vi "ROI.vi"(0 "input cluster":T2) -> (1 "Acquired Buffer Number":u32, 2 "Output First-call":bool=TRUE, 3 "Output ROI Array":dbl[][](array[numeric]))   [LabVIEW 2010]
uses:
  <vilib>/userDefined/High Color/IMAQdx.ctl
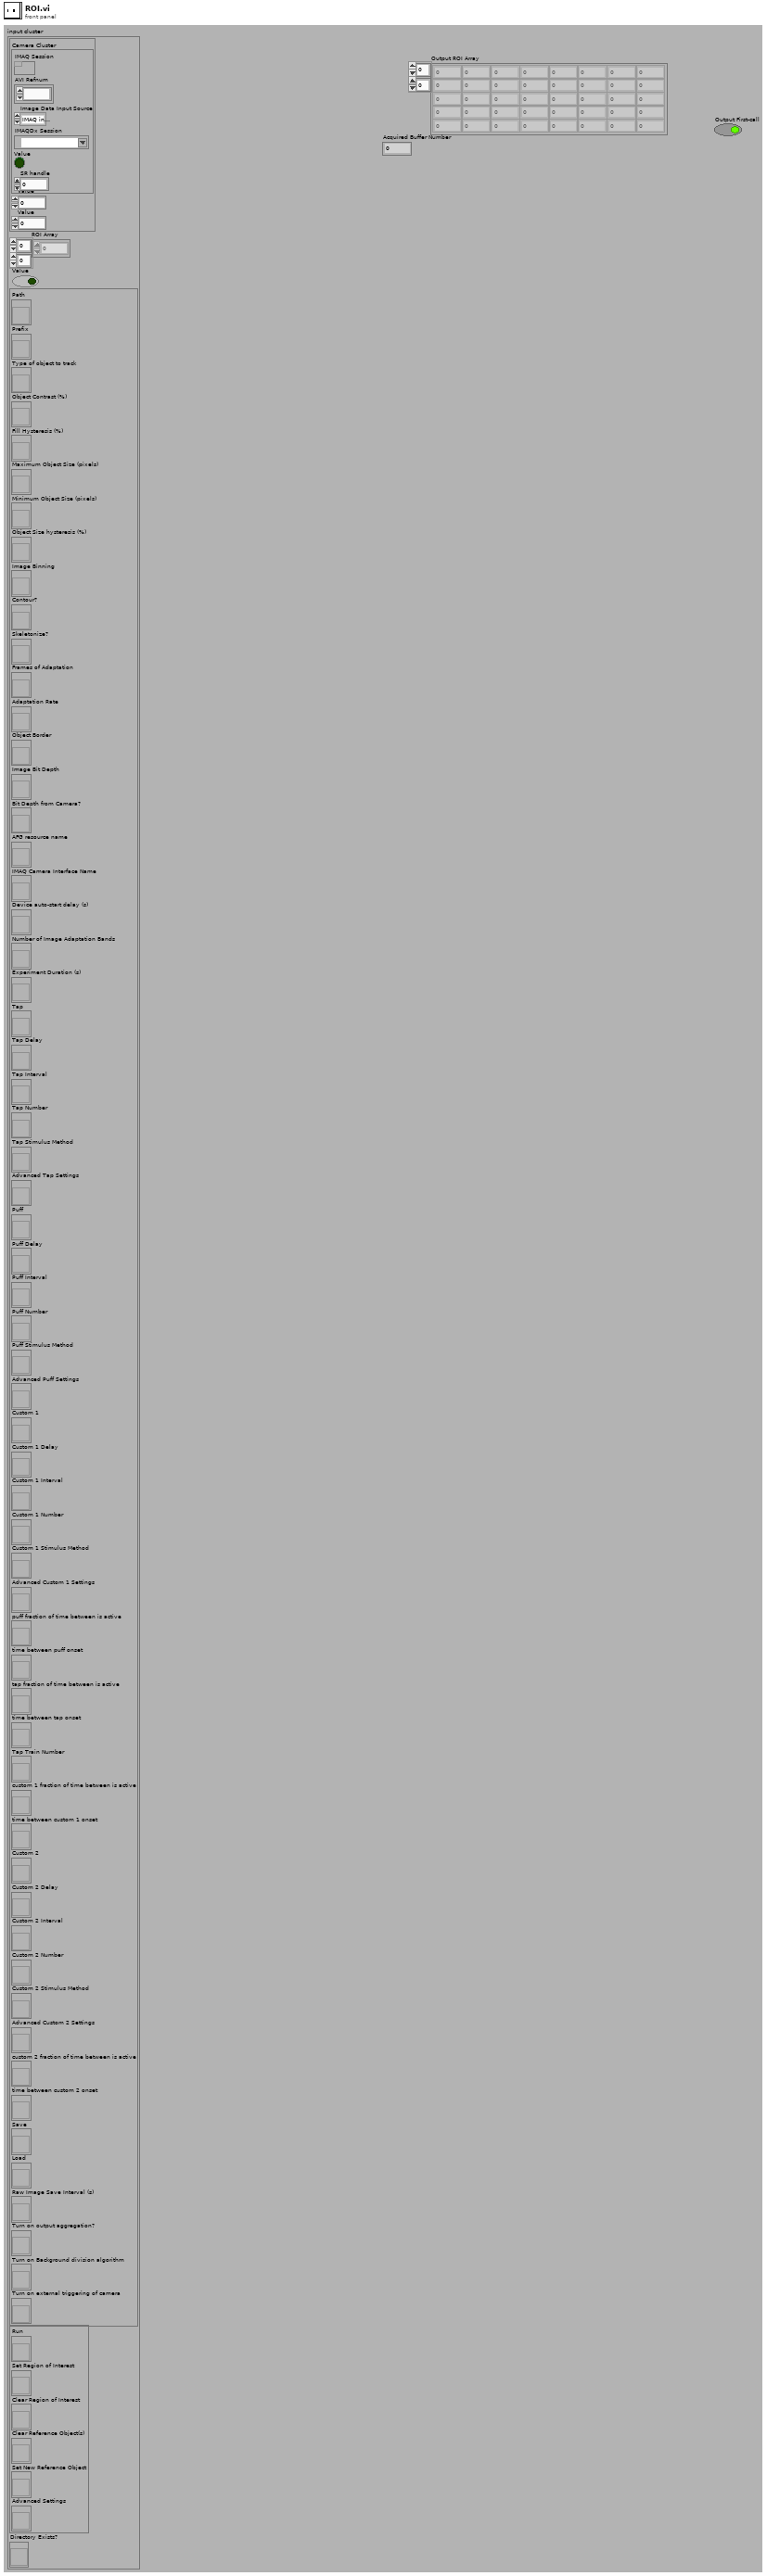
[diagram p1: front panel]
types:
  T1 = typedef "IMAQdx.ctl" = refnum<k21>
  T2 = cluster{cluster{"Camera Cluster":cluster{"IMAQ Session":refnum<k11>, "AVI Refnum":refnum<k1>, "Image Data Input Source":enum32{"IMAQ interface", "IMAQdx interface", "AVI file", "MMF File"}, "IMAQDx Session":T1, "Value":bool, "SR handle":u32}, "Value":i32, "Value":i32}, "ROI Array":dbl[][], "Value":bool, cluster{"Path":refnum<vi>, "Prefix":refnum<vi>, "Type of object to track":refnum<vi>, "Object Contrast (%)":refnum<vi>, "Fill Hysteresis (%)":refnum<vi>, "Maximum Object Size (pixels)":refnum<vi>, "Minimum Object Size (pixels)":refnum<vi>, "Object Size hysteresis (%)":refnum<vi>, "Image Binning":refnum<vi>, "Contour?":refnum<vi>, "Skeletonize?":refnum<vi>, "Frames of Adaptation":refnum<vi>, "Adaptation Rate":refnum<vi>, "Object Border":refnum<vi>, "Image Bit Depth":refnum<vi>, "Bit Depth from Camera?":refnum<vi>, "AFG resource name":refnum<vi>, "IMAQ Camera Interface Name":refnum<vi>, "Device auto-start delay (s)":refnum<vi>, "Number of Image Adaptation Bands":refnum<vi>, "Experiment Duration (s)":refnum<vi>, "Tap":refnum<vi>, "Tap Delay":refnum<vi>, "Tap Interval":refnum<vi>, "Tap Number":refnum<vi>, "Tap Stimulus Method":refnum<vi>, "Advanced Tap Settings":refnum<vi>, "Puff":refnum<vi>, "Puff Delay":refnum<vi>, "Puff Interval":refnum<vi>, "Puff Number":refnum<vi>, "Puff Stimulus Method":refnum<vi>, "Advanced Puff Settings":refnum<vi>, "Custom 1":refnum<vi>, "Custom 1 Delay":refnum<vi>, "Custom 1 Interval":refnum<vi>, "Custom 1 Number":refnum<vi>, "Custom 1 Stimulus Method":refnum<vi>, "Advanced Custom 1 Settings":refnum<vi>, "puff fraction of time between is active":refnum<vi>, "time between puff onset":refnum<vi>, "tap fraction of time between is active":refnum<vi>, "time between tap onset":refnum<vi>, "Tap Train Number":refnum<vi>, "custom 1 fraction of time between is active":refnum<vi>, "time between custom 1 onset":refnum<vi>, "Custom 2":refnum<vi>, "Custom 2 Delay":refnum<vi>, "Custom 2 Interval":refnum<vi>, "Custom 2 Number":refnum<vi>, "Custom 2 Stimulus Method":refnum<vi>, "Advanced Custom 2 Settings":refnum<vi>, "custom 2 fraction of time between is active":refnum<vi>, "time between custom 2 onset":refnum<vi>, "Save":refnum<vi>, "Load":refnum<vi>, "Raw Image Save Interval (s)":refnum<vi>, "Turn on output aggregation?":refnum<vi>, "Turn on Background division algorithm":refnum<vi>, "Turn on external triggering of camera":refnum<vi>}, cluster{"Run":refnum<vi>, "Set Region of Interest":refnum<vi>, "Clear Region of Interest":refnum<vi>, "Clear Reference Object(s)":refnum<vi>, "Set New Reference Object":refnum<vi>, "Advanced Settings":refnum<vi>}, "Directory Exists?":refnum<vi>}
  T3 = cluster{"Camera Cluster":cluster{"IMAQ Session":refnum<k11>, "AVI Refnum":refnum<k1>, "Image Data Input Source":enum32{"IMAQ interface", "IMAQdx interface", "AVI file", "MMF File"}, "IMAQDx Session":T1, "Value":bool, "SR handle":u32}, "Value":i32, "Value":i32}
  T4 = cluster{"Path":refnum<vi>, "Prefix":refnum<vi>, "Type of object to track":refnum<vi>, "Object Contrast (%)":refnum<vi>, "Fill Hysteresis (%)":refnum<vi>, "Maximum Object Size (pixels)":refnum<vi>, "Minimum Object Size (pixels)":refnum<vi>, "Object Size hysteresis (%)":refnum<vi>, "Image Binning":refnum<vi>, "Contour?":refnum<vi>, "Skeletonize?":refnum<vi>, "Frames of Adaptation":refnum<vi>, "Adaptation Rate":refnum<vi>, "Object Border":refnum<vi>, "Image Bit Depth":refnum<vi>, "Bit Depth from Camera?":refnum<vi>, "AFG resource name":refnum<vi>, "IMAQ Camera Interface Name":refnum<vi>, "Device auto-start delay (s)":refnum<vi>, "Number of Image Adaptation Bands":refnum<vi>, "Experiment Duration (s)":refnum<vi>, "Tap":refnum<vi>, "Tap Delay":refnum<vi>, "Tap Interval":refnum<vi>, "Tap Number":refnum<vi>, "Tap Stimulus Method":refnum<vi>, "Advanced Tap Settings":refnum<vi>, "Puff":refnum<vi>, "Puff Delay":refnum<vi>, "Puff Interval":refnum<vi>, "Puff Number":refnum<vi>, "Puff Stimulus Method":refnum<vi>, "Advanced Puff Settings":refnum<vi>, "Custom 1":refnum<vi>, "Custom 1 Delay":refnum<vi>, "Custom 1 Interval":refnum<vi>, "Custom 1 Number":refnum<vi>, "Custom 1 Stimulus Method":refnum<vi>, "Advanced Custom 1 Settings":refnum<vi>, "puff fraction of time between is active":refnum<vi>, "time between puff onset":refnum<vi>, "tap fraction of time between is active":refnum<vi>, "time between tap onset":refnum<vi>, "Tap Train Number":refnum<vi>, "custom 1 fraction of time between is active":refnum<vi>, "time between custom 1 onset":refnum<vi>, "Custom 2":refnum<vi>, "Custom 2 Delay":refnum<vi>, "Custom 2 Interval":refnum<vi>, "Custom 2 Number":refnum<vi>, "Custom 2 Stimulus Method":refnum<vi>, "Advanced Custom 2 Settings":refnum<vi>, "custom 2 fraction of time between is active":refnum<vi>, "time between custom 2 onset":refnum<vi>, "Save":refnum<vi>, "Load":refnum<vi>, "Raw Image Save Interval (s)":refnum<vi>, "Turn on output aggregation?":refnum<vi>, "Turn on Background division algorithm":refnum<vi>, "Turn on external triggering of camera":refnum<vi>}
  T5 = cluster{"Run":refnum<vi>, "Set Region of Interest":refnum<vi>, "Clear Region of Interest":refnum<vi>, "Clear Reference Object(s)":refnum<vi>, "Set New Reference Object":refnum<vi>, "Advanced Settings":refnum<vi>}
  T6 = cluster{"IMAQ Session":refnum<k11>, "AVI Refnum":refnum<k1>, "Image Data Input Source":enum32{"IMAQ interface", "IMAQdx interface", "AVI file", "MMF File"}, "IMAQDx Session":T1, "Value":bool, "SR handle":u32}
  T7 = cluster{"Camera Cluster":cluster{"IMAQ Session":refnum<k11>, "AVI Refnum":refnum<k1>, "Image Data Input Source":enum32{"IMAQ interface", "IMAQdx interface", "AVI file", "MMF File"}, "IMAQDx Session":T1, "Value":bool, "SR handle":u32}, "Value":i32}
  T8 = cluster{cluster{"Camera Cluster":cluster{"IMAQ Session":refnum<k11>, "AVI Refnum":refnum<k1>, "Image Data Input Source":enum32{"IMAQ interface", "IMAQdx interface", "AVI file", "MMF File"}, "IMAQDx Session":T1, "Value":bool, "SR handle":u32}, "Value":i32}, "Value":i32, "Output ROI Array":dbl[][]}
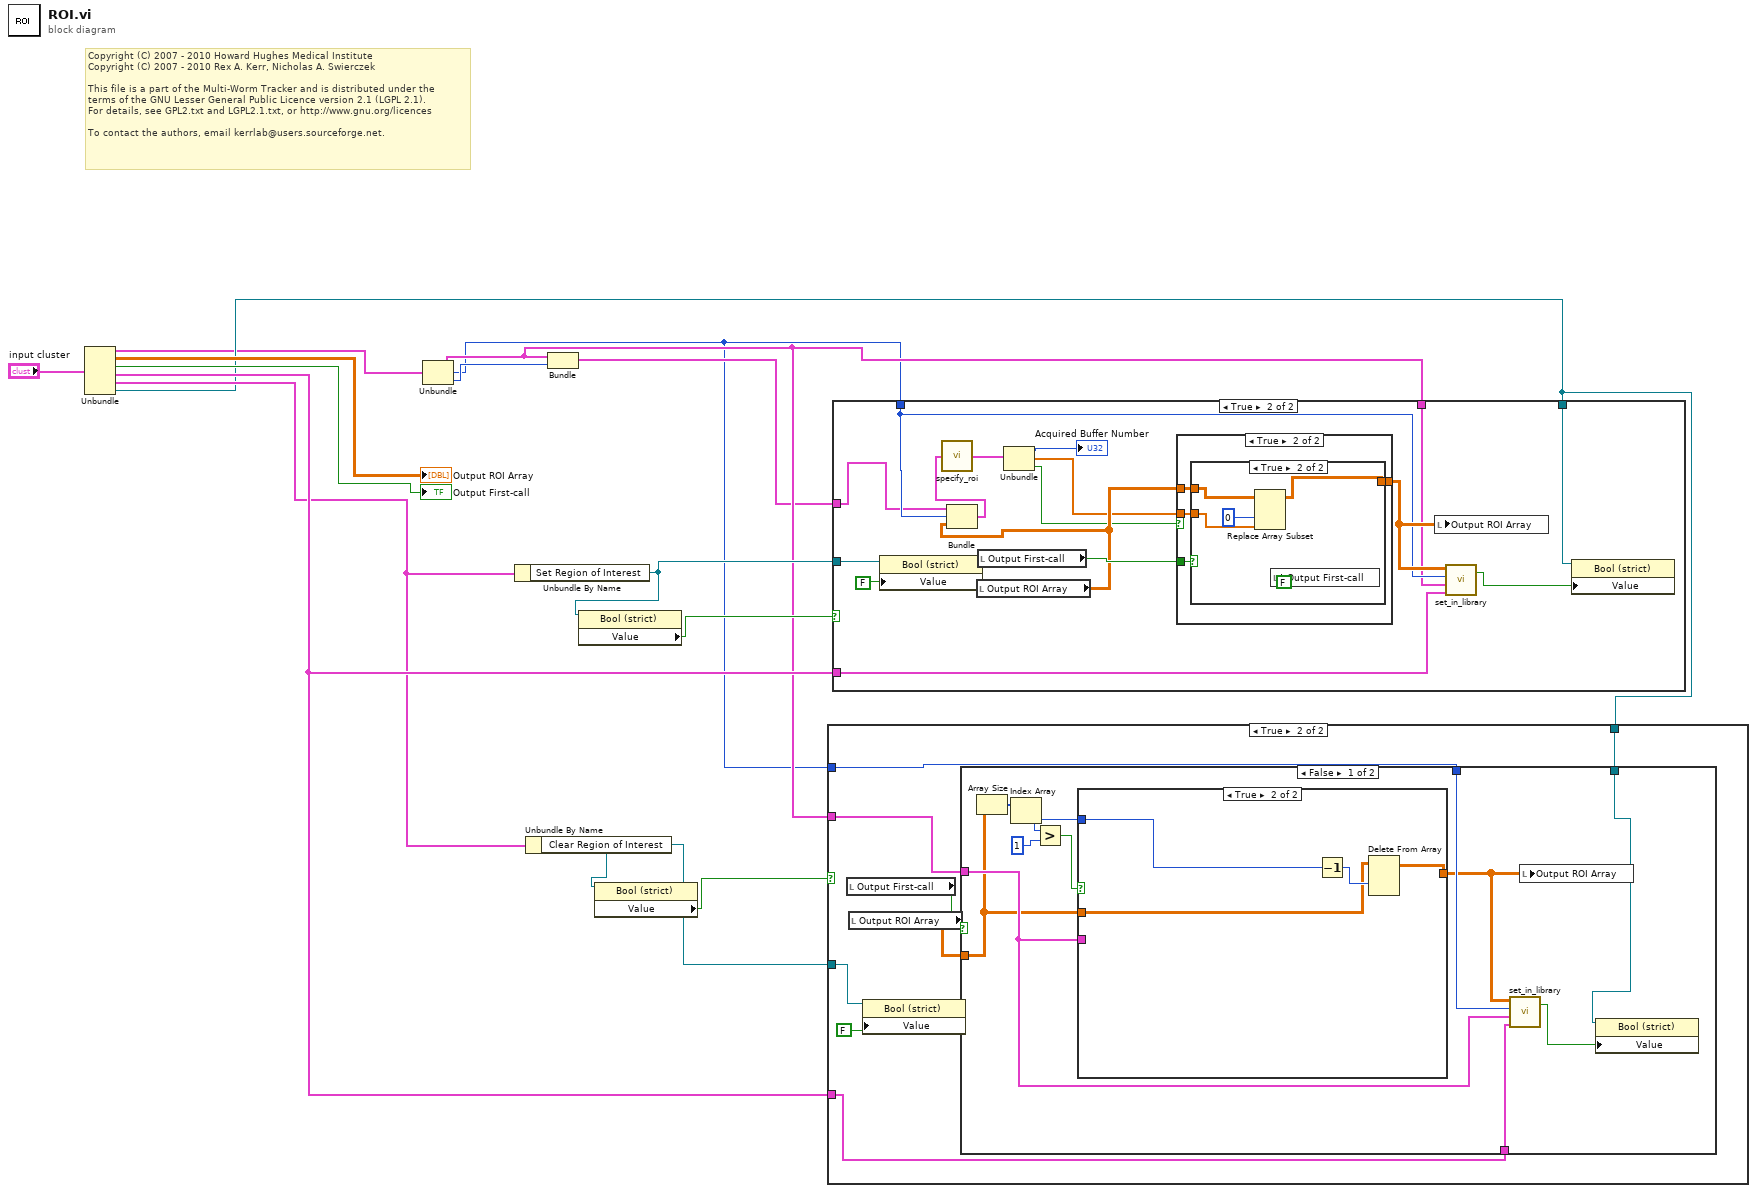
[diagram p0: block diagram]
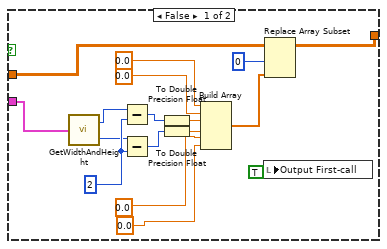
[diagram p3: hidden frame]
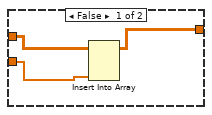
[diagram p7: hidden frame]
diagram:
  # "Copyright (C) 2007 - 2010 Howard Hughes Medical Institute\nCopyright (C) 2007 - 2010 Rex A. Kerr, Nicholas A. Swierczek\n \nThis file is a part of the Multi-Worm Tracker and is distributed under the\nterms of the GNU Lesser General Public Licence version 2.1 (LGPL 2.1).\nFor details, see GPL2.txt and LGPL2.1.txt, or http://www.gnu.org/licences\n \nTo contact the authors, email kerrlab@users.sourceforge.net."
  n1 = Unbundle("input cluster") -> (w6:T3, "ROI Array"=→"Output ROI Array":dbl[][], "Value"=→"Output First-call":bool, w9:T4, w8:T5, "Directory Exists?"=w7:refnum<vi>)
  n2 = Unbundle(w6) -> ("Camera Cluster"=w4:T6, "Value"=w2:i32, "Value"=w5:i32)
  n3 = Unbundle By Name(w8) -> ("Set Region of Interest"=w15:refnum<vi>)
  n4 = Unbundle By Name(w8) -> ("Clear Region of Interest"=w12:refnum<vi>)
  n5 = Bundle("Camera Cluster"=w4, "Value"=w5) -> (w3:T7)  [unwired: 1 in]
  n6 = property class="Bool (strict)"(reference=w15) -> ("Value"=w14:bool)  [unwired: 1 in, 2 out]
  n7 = property class="Bool (strict)"(reference=w12) -> ("Value"=w13:bool)  [unwired: 1 in, 2 out]
  n8 = case shown="True" w13 {
    tunnel: w12 -> [_ w17]
    tunnel: w4 -> [_ w21]
    tunnel: w9 -> [_ w20]
    tunnel: w2 -> [_ w19]
    tunnel: w7 -> [_ w18]
    frame False {
    }
    frame True {
      n9 = local read "Output First-call"() -> (w23:bool)
      n10 = local read "Output ROI Array"() -> (w22:dbl[][])
      n11 = property class="Bool (strict)"(reference=w17, "Value"=FALSE ("OK Button")) -> ()  [unwired: 1 in, 2 out]
      n12 = case shown="False" w23 {
        tunnel: w22 -> [w28 _]
        tunnel: w21 -> [w30 _]
        tunnel: w20 -> [w32 _]
        tunnel: w19 -> [w31 _]
        tunnel: w18 -> [w25 _]
        frame False {
          n13 = Array Size(array=w28) -> (size(s)=w29:i32[])
          n14 = Index Array(array=w29) -> (element=w27:i32)  [unwired: 1 in]
          n15 = Greater?(x=w27, y=1) -> (0:w33:bool)
          n16 = case shown="True" w33 {
            tunnel: [w51 w53] -> w26
            tunnel: w30 -> [w37 _]
            tunnel: w28 -> [w43 w54]
            tunnel: w27 -> [_ w52]
            frame False {
              w38 = u32 2 ("y")
              n17 = call "GetWidthAndHeight.vi"("Camera Cluster"=w37) -> ("Width"=w36:u32, "Height"=w35:u32)
              n18 = Subtract(x=w36, y=w38) -> (x-y=w41:u32)
              n19 = Subtract(x=w35, y=w38) -> (x-y=w42:u32)
              n20 = To Double Precision Float(number=w41) -> (double precision float=w48:dbl)
              n21 = To Double Precision Float(number=w42) -> (double precision float=w49:dbl)
              n22 = Build Array(0.0, 0.0, w48, w49, 0.0, 0.0) -> (w45:dbl[])
              n23 = local write "Output First-call"(TRUE ("First-call")) -> ()
              n24 = Replace Array Subset(array=w43, new element=w45, index (row)=0) -> (w51:dbl[][])  [unwired: 1 in]
            }
            frame True {
              n25 = Decrement(x=w52) -> (x-1=w55:i32)
              n26 = Delete From Array(array=w54, index (row)=w55) -> (array with subset deleted=w53:dbl[][])  [unwired: 2 in, 1 out]
            }
          }
          n27 = call "set_in_library.vi"("Cluster"=w32, "Camera Cluster"=w30, "Tracker Handle"=w31, "Array"=w26) -> ("Directory Exists?"=w24:bool)  [unwired: 1 out]
          n28 = local write "Output ROI Array"(w26) -> ()
          n29 = property class="Bool (strict)"(reference=w25, "Value"=w24) -> ()  [unwired: 1 in, 2 out]
        }
        frame True {
          # "Do nothing"
        }
      }
    }
  }
  n30 = case shown="True" w14 {
    tunnel: w3 -> [_ w60]
    tunnel: w2 -> [_ w64]
    tunnel: w15 -> [_ w66]
    tunnel: w9 -> [_ w70]
    tunnel: w7 -> [_ w68]
    tunnel: w4 -> [_ w63]
    frame False {
    }
    frame True {
      n31 = property class="Bool (strict)"(reference=w66, "Value"=FALSE ("OK Button")) -> ()  [unwired: 1 in, 2 out]
      n32 = local read "Output ROI Array"() -> (w62:dbl[][])
      n33 = Bundle(w60, "Value"=w64, "Output ROI Array"=w62) -> (w56:T8)  [unwired: 1 in]
      n34 = call "specify_roi.vi"("input cluster"=w56) -> ("output cluster"=w59:cluster{"Value":i32, dbl[], "Set":bool})
      n35 = local read "Output First-call"() -> (w71:bool)
      n36 = Unbundle(w59) -> ("Value"=→"Acquired Buffer Number":i32, w57:dbl[], "Set"=w61:bool)
      n37 = case shown="True" w61 {
        tunnel: w57 -> [_ w76]
        tunnel: w71 -> [_ w75]
        tunnel: [w72 w74] -> w69
        tunnel: w62 -> [w72 w73]
        frame False {
        }
        frame True {
          n38 = case shown="True" w75 {
            tunnel: w76 -> [w79 w82]
            tunnel: [w77 w84] -> w74
            tunnel: w73 -> [w78 w80]
            frame False {
              n39 = Insert Into Array(array=w78, new element=w79) -> (w77:dbl[][])  [unwired: 2 in]
            }
            frame True {
              n40 = Replace Array Subset(array=w80, new element=w82, index (row)=0) -> (w84:dbl[][])  [unwired: 1 in]
              n41 = local write "Output First-call"(FALSE ("First-call")) -> ()
            }
          }
        }
      }
      n42 = local write "Output ROI Array"(w69) -> ()
      n43 = call "set_in_library.vi"("Cluster"=w70, "Camera Cluster"=w63, "Tracker Handle"=w64, "Array"=w69) -> ("Directory Exists?"=w67:bool)  [unwired: 1 out]
      n44 = property class="Bool (strict)"(reference=w68, "Value"=w67) -> ()  [unwired: 1 in, 2 out]
    }
  }
